vi "Send.vi"(8 "error in (no error)":errorcluster, 10 "Message":T1, 11 "Queue Name":string) -> (0 "error out":errorcluster)   [LabVIEW 2019, in "Messaging.lvlib"]
doc: "Sends the Message to the queue specified by Queue Name. If the named queue does not exist, the message is not sent.\n\nIf the named queue does exist, the queue reference is stored in this VI and reused."
uses:
  Messaging.lvlib
  Message Cluster.ctl
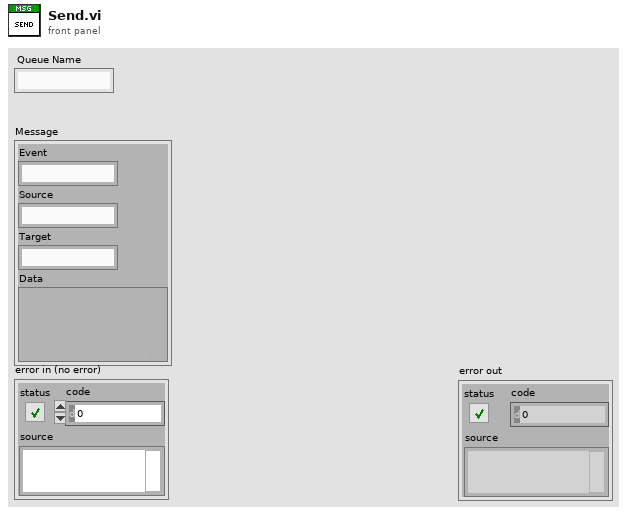
[diagram p1: front panel]
types:
  T1 = typedef "Messaging.lvlib/Message Cluster.ctl" = cluster{"Event":string, "Source":string, "Target":string, "Data":variant}
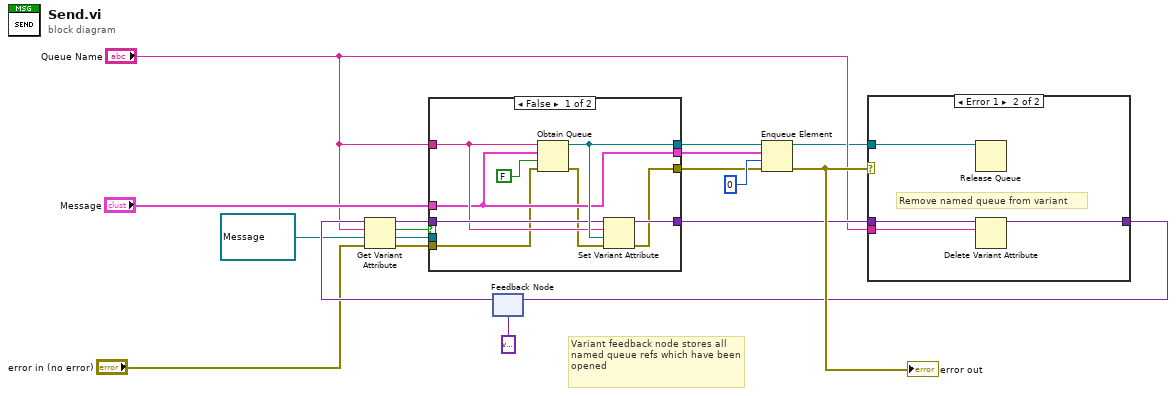
[diagram p0: block diagram]
diagram:
  # "Variant feedback node stores all named queue refs which have been opened"
  n1 = feedback #1(variant) -> (w14:variant)
  n2 = Get Variant Attribute(Variant=w14, name="Queue Name", default value (empty Variant)=refnum<queue> refnum ("queue out"), error in="error in (no error)") -> (duplicate Variant=w9:variant, found=w12:bool, value=w11:refnum<queue>, error out=w7:errorcluster)
  n3 = case shown="False" w12 {
    tunnel: "Message" -> [w22 w30]
    tunnel: [w26 w31] -> w16
    tunnel: "Queue Name" -> [w23 _]
    tunnel: w11 -> [_ w31]
    tunnel: [w22 w30] -> w10
    tunnel: [w25 w29] -> w4
    tunnel: w9 -> [w24 w29]
    tunnel: [w20 w28] -> w8
    tunnel: w7 -> [w19 w28]
    frame False {
      n4 = Obtain Queue(name (unnamed)=w23, element data type=w22, create if not found? (T)=FALSE, error in (no error)=w19) -> (queue out=w26:refnum<queue>, error out=w21:errorcluster)  [unwired: 1 in, 1 out]
      n5 = Set Variant Attribute(Variant=w24, name=w23, value=w26, error in=w21) -> (Variant out=w25:variant, error out=w20:errorcluster)  [unwired: 1 out]
    }
    frame True {
    }
  }
  n6 = Enqueue Element(queue=w16, element=w10, timeout in ms (-1)=0, error in (no error)=w8) -> (queue out=w1:refnum<queue>, error out=w5:errorcluster)  [unwired: 1 out]
  "error out" <- w5
  n7 = case shown="Error 1" w5 {
    tunnel: w4 -> [w32 w36]
    tunnel: [w32 w35] -> w3
    tunnel: "Queue Name" -> [_ w34]
    tunnel: w1 -> [_ w33]
    frame #0 {
    }
    frame #1 {
      # "Remove named queue from variant"
      n8 = Release Queue(queue=w33) -> ()  [unwired: 2 in, 3 out]
      n9 = Delete Variant Attribute(6:w34, 7:w36) -> (3:w35:variant)  [unwired: 1 in, 2 out]
    }
  }
  n10 = feedback-in #1(w3) -> ()
